vi "Fire User Event - Stop.vi"(8 "error in (no error)":errorcluster, 11 "User Event - Stop":refnum<user-event>) -> (0 "error out":errorcluster)   [LabVIEW 2019, in "User Event - Stop.lvlib"]
doc: "Send the Stop event to stop the Event Handling Loop."
uses:
  User Event - Stop.lvlib
  <vilib>/event_ctls.llb/usereventprio.ctl
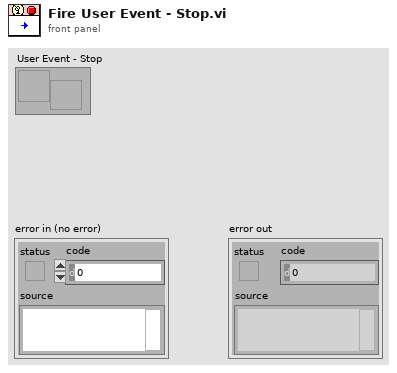
[diagram p1: front panel]
types:
  T1 = typedef "usereventprio.ctl" = enum32{"high priority", "normal priority"}
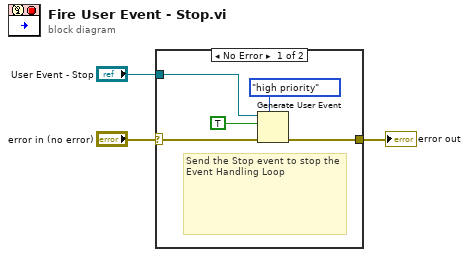
[diagram p0: block diagram]
diagram:
  n1 = case shown="No Error" "error in (no error)" {
    selector: "error in (no error)" -> [w5 w9]
    tunnel: [w7 w9] -> w3
    tunnel: "User Event - Stop" -> [w6 _]
    frame No Error {
      # "Send the Stop event to stop the Event Handling Loop"
      n2 = Generate User Event(priority (normal)=usereventprio."high priority", user event=w6, event data cluster=TRUE ("event data"), error in=w5) -> (error out=w7:errorcluster)  [unwired: 1 out]
    }
    frame Error {
    }
  }
  "error out" <- w3
